vi "clone.vi"(0 "reference":refnum<class "ClassRelationshipEdge.lvclass">, 5 "error in (no error)":errorcluster) -> (14 "reference out":refnum<class "ClassRelationshipEdge.lvclass">, 15 "clonedEdge":refnum<class "AbstractEdge.lvclass">, 19 "error out":errorcluster)   [LabVIEW 2012, in "ClassRelationshipEdge.lvclass"]
doc: "Clone"
uses:
  <resource>/Framework/Providers/Open_GDS/UML/ClassRelationshipEdge_class/ClassRelationshipEdge.lvclass
  <resource>/Framework/Providers/Open_GDS/UML/AbstractEdge_class/AbstractEdge.lvclass
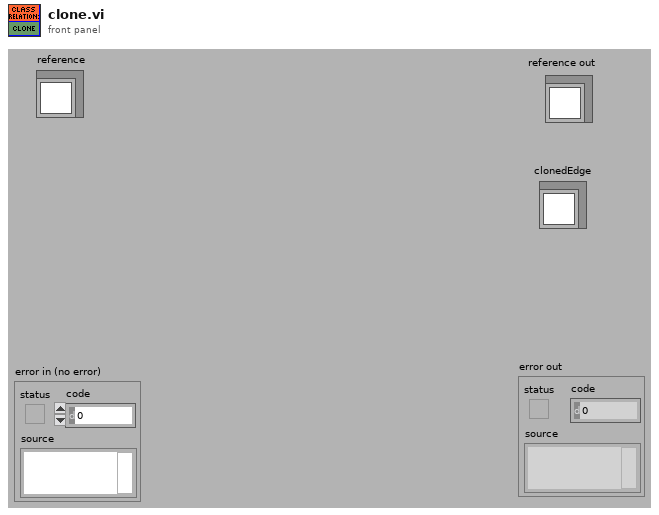
[diagram p1: front panel]
types:
  T1 = typedef "ClassRelationshipEdge.lvclass/ObjectAttributes.ctl" = cluster{"Base class":T2, "bentStyleRef":refnum<class "BentStyle.lvclass">, "startConnectionOffset":cluster{"x":i32, "y":i32}, "endConnectionOffset":cluster{"x":i32, "y":i32}, "MidLineOffset":cluster{"x":i32, "y":i32}, "DepClass":T6}
  T2 = typedef "SegmentedLineEdge.lvclass/ObjectAttributes.ctl" = cluster{"Base class":T3, "lineStyle":refnum<class "LineStyle.lvclass">, "startArrowHead":refnum<class "ArrowHead.lvclass">, "endArrowHead":refnum<class "ArrowHead.lvclass">, "startLabel":string, "midLabel":string, "endLabel":string, "MidLabelOffset":T5, "SplitWire":bool}
  T3 = typedef "GeneralPathEdge.lvclass/ObjectAttributes.ctl" = cluster{"Base class":T4}
  T4 = typedef "AbstractEdge.lvclass/ObjectAttributes.ctl" = cluster{"start":refnum<class "AbstractNode.lvclass">, "end":refnum<class "AbstractNode.lvclass">}
  T5 = typedef "Point Point2D.ctl" = cluster{"x":dbl, "y":dbl}
  T6 = typedef "ReversedEngineering_ViDependencyDetailsType.ctl" = cluster{"ThisVIs/Ctls":path[], "Dependent_VIs/Ctls":path[]}
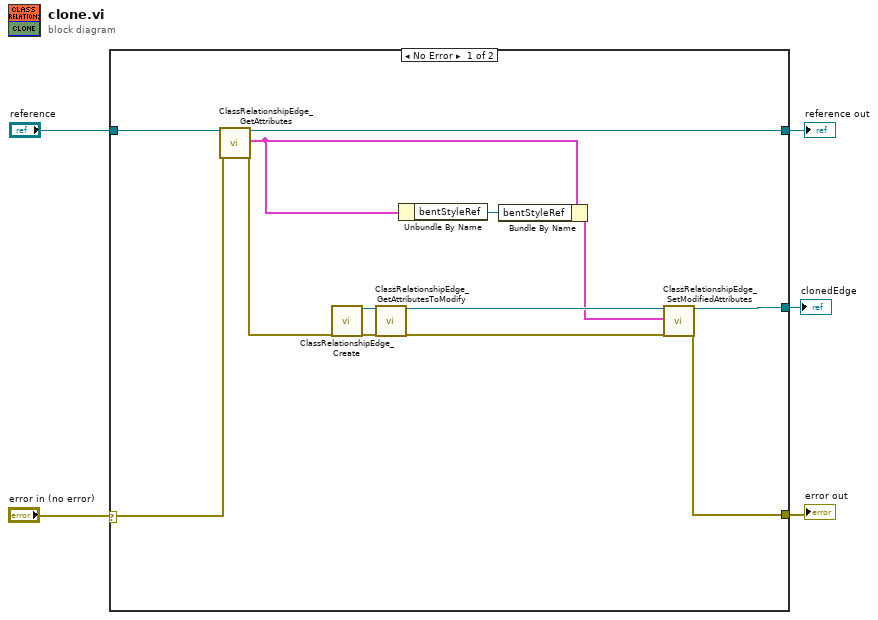
[diagram p0: block diagram]
diagram:
  n1 = case shown="No Error" "error in (no error)" {
    selector: "error in (no error)" -> [w10 w19]
    tunnel: "reference" -> [w18 w20]
    tunnel: [w17 w19] -> w4
    tunnel: [w8 w20] -> w3
    tunnel: [w16 _] -> w1
    frame No Error {
      n2 = call <resource>:"ClassRelationshipEdge_GetAttributes.vi"("reference in"=w18, "error in (no error)"=w10) -> ("reference out"=w8:refnum<class "ClassRelationshipEdge.lvclass">, "Attributes"=w9:T1, "error out"=w7:errorcluster)  [unwired: 15 out]
      n3 = call <resource>:"ClassRelationshipEdge_Create.vi"("error in (no error)"=w7) -> ("reference out"=w6:refnum<class "ClassRelationshipEdge.lvclass">, "error out"=w15:errorcluster)  [unwired: 16 in, 1 out]
      n4 = call <resource>:"ClassRelationshipEdge_GetAttributesToModify.vi"("reference in"=w6, "error in (no error)"=w15) -> ("reference out"=w14:refnum<class "ClassRelationshipEdge.lvclass">, "error out"=w13:errorcluster)  [unwired: 1 in, 15 out]
      n5 = Unbundle By Name(w9) -> ("bentStyleRef"=w11:refnum<class "BentStyle.lvclass">)
      n6 = Bundle By Name(cluster=w9, "bentStyleRef"=w11) -> (w12:T1)
      n7 = call <resource>:"ClassRelationshipEdge_SetModifiedAttributes.vi"("reference in"=w14, "Attributes"=w12, "error in (no error)"=w13) -> ("reference out"=w16:refnum<class "ClassRelationshipEdge.lvclass">, "error out"=w17:errorcluster)  [unwired: 3 in, 12 out]
    }
    frame Error {
    }
  }
  "reference out" <- w3
  "error out" <- w4
  "clonedEdge" <- w1
